vi "Clear Limit Test Results.vi"(0 "VISA resource name":refnum<visa-resource-name>, 5 "Function":u16(ring) items=["Voltage: DC", "Voltage: AC", "Current: DC", "Current: AC", "2W Resistance", "4W Resistance", "Diode", "Capacitance", "Temperature", "Continuity", "Frequency", "Period", "Ratio", "Digitize Voltage", "Digitize Current"], 7 "Limit Test Number":u16=1 min=1 max=2 step=1, 11 "error in (no error)":errorcluster) -> (4 "VISA resource name out":refnum<visa-resource-name>, 15 "error out":errorcluster)   [LabVIEW 2016, in "Keithley DMM7510.lvlib"]
doc: "This command clears the results of the limit test."
uses:
  Keithley DMM7510.lvlib
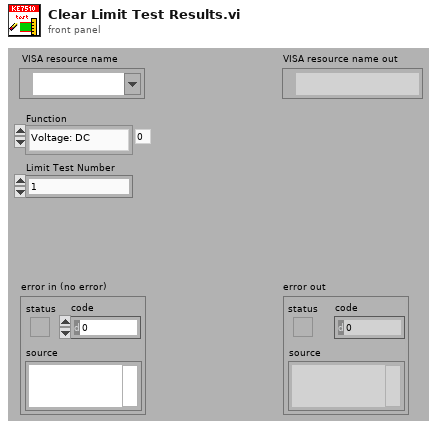
[diagram p1: front panel]
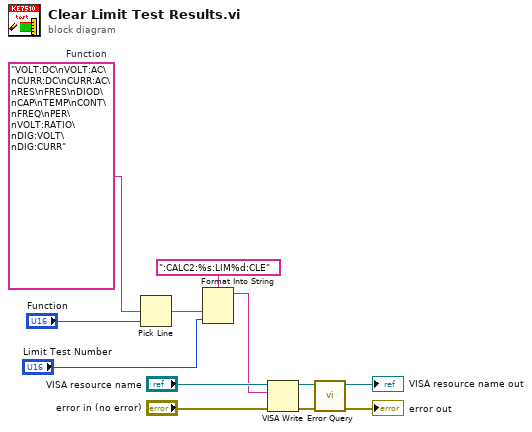
[diagram p0: block diagram]
diagram:
  w3 = "VOLT:DC\nVOLT:AC\nCURR:DC\nCURR:AC\nRES\nFRES\nDIOD\nCAP\nTEMP\nCONT\nFREQ\nPER\nVOLT:RATIO\nDIG:VOLT\nDIG:CURR"  # Function
  n1 = Pick Line(multi-line string=w3, line index="Function") -> (output string=w4:string)  [unwired: 1 out]
  n2 = Format Into String(format string=":CALC2:%s:LIM%d:CLE", w4, "Limit Test Number") -> (resulting string=w5:string)  [unwired: 2 in, 1 out]
  n3 = VISA Write(VISA resource name="VISA resource name", write buffer=w5, error in (no error)="error in (no error)") -> (VISA resource name out=w8:refnum<visa-resource-name>, error out=w7:errorcluster)  [unwired: 1 out]
  n4 = call "Error Query.vi"("error in (no error)"=w7, "VISA resource name"=w8) -> ("error out"=→"error out":errorcluster, "VISA resource name out"=→"VISA resource name out":refnum<visa-resource-name>)  [unwired: 8 out]
